vi "CMN_Non-standard-testpath.vi"(8 "error in":errorcluster, 10 "ModuleName":string, 11 "caller Path":path) -> (0 "error out":errorcluster, 2 "ConfigFile":path)   [LabVIEW 2016]
panel:
  out "path":path
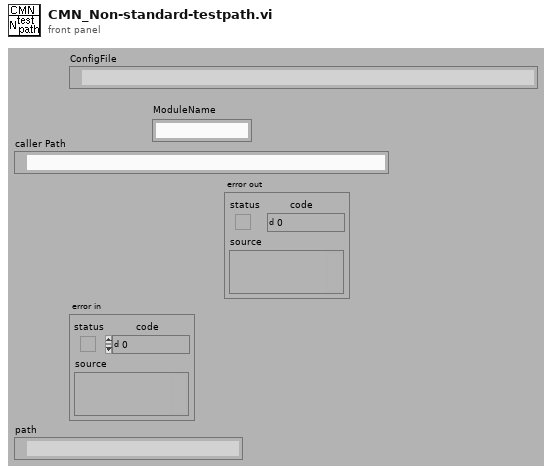
[diagram p1: front panel]
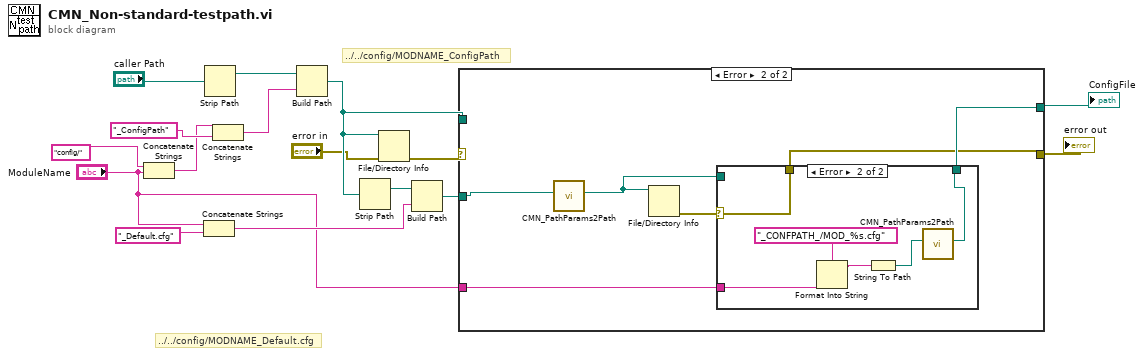
[diagram p0: block diagram]
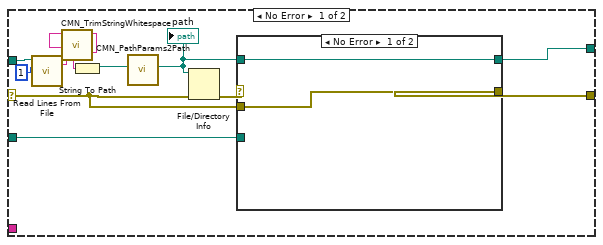
[diagram p2: hidden frame]
diagram:
  # "../../config/MODNAME_ConfigPath"
  # "../../config/MODNAME_Default.cfg"
  n1 = Concatenate Strings("config/", "ModuleName") -> (w8:string)
  n2 = Concatenate Strings("ModuleName", "_Default.cfg" ("string")) -> (w11:string)
  n3 = Strip Path(path="caller Path") -> (stripped path=w4:path)  [unwired: 1 out]
  n4 = Concatenate Strings(w8, "_ConfigPath" ("string")) -> (w10:string)
  n5 = Build Path(base path=w4, name or relative path=w10) -> (appended path=w9:path)
  n6 = Strip Path(path=w9) -> (stripped path=w14:path)  [unwired: 1 out]
  n7 = File/Directory Info(path=w9, error in="error in") -> (error out=w15:errorcluster)  [unwired: 6 out]
  n8 = Build Path(base path=w14, name or relative path=w11) -> (appended path=w7:path)
  n9 = case shown="Error" w15 {
    selector: w15 -> [w22 _]
    tunnel: w9 -> [w27 _]
    tunnel: [w25 w34] -> w2
    tunnel: w7 -> [w24 w37]
    tunnel: [w23 w33] -> w6
    tunnel: "ModuleName" -> [_ w32]
    frame No Error {
      n10 = call <vilib>:"Read Lines From File.vi"("file path (dialog if empty)"=w27, "number of lines (all:-1)"=1) -> ("line string"=w20:string)  [unwired: 7 out]
      n11 = call "CMN_TrimStringWhitespace.vi"("string"=w20) -> ("trimmed string"=w19:string)  [unwired: 1 in, 8 out]
      n12 = String To Path(string=w19) -> (path=w18:path)
      n13 = call "CMN_PathParams2Path.vi"("Path In"=w18) -> ("Path out"=w17:path)  [unwired: 2 in, 8 out]
      "path" <- w17
      n14 = File/Directory Info(path=w17, error in=w22) -> (error out=w26:errorcluster)  [unwired: 6 out]
      n15 = case shown="No Error" w26 {
        tunnel: w17 -> [w29 _]
        tunnel: [w29 w31] -> w25
        tunnel: w24 -> [_ w31]
        tunnel: [w28 w30] -> w23
        tunnel: w22 -> [w28 w30]
        frame No Error {
        }
        frame Error {
        }
      }
    }
    frame Error {
      n16 = call "CMN_PathParams2Path.vi"("Path In"=w37) -> ("Path out"=w35:path)  [unwired: 2 in, 8 out]
      n17 = File/Directory Info(path=w35) -> (error out=w36:errorcluster)  [unwired: 1 in, 6 out]
      n18 = case shown="Error" w36 {
        selector: w36 -> [w39 w45]
        tunnel: w35 -> [w38 _]
        tunnel: [w38 w40] -> w34
        tunnel: [w39 w45] -> w33
        tunnel: w32 -> [_ w43]
        frame No Error {
        }
        frame Error {
          n19 = Format Into String(format string="_CONFPATH_/MOD_%s.cfg", w43) -> (resulting string=w42:string)  [unwired: 2 in, 1 out]
          n20 = String To Path(string=w42) -> (path=w41:path)
          n21 = call "CMN_PathParams2Path.vi"("Path In"=w41) -> ("Path out"=w40:path)  [unwired: 2 in, 8 out]
        }
      }
    }
  }
  "error out" <- w6
  "ConfigFile" <- w2
